vi "DefenderPenalty.vi"(6 "N atacantes":u32[](array[numeric]), 10 "Total de n \natacantes":i32, 11 "Robot in":T1={"id"=0, "function"=enum."Attacker", "x"=0.0, "y"=0.0, "orientation"=0.0, "v_tangent"=0.0, "v_normal"=0.0, "v_ang"=0.0, "kick_x"=0.0, "kick_z"=0.0, "dribble"=FALSE, "Timestamp"=timestamp(0 s since 1904-01-01), "estimatives"={"est_v_tangent"=0.0, "est_v_normal"=0.0, "est_vx"=0.0, "est_vy"=0.0, "Pos Robot Est"=[]}, "dest_x_kick"=0.0, "dest_y_kick"=0.0, "Gap Coord"=[], "States"=enum."GoToTangent", "Path "=[], "Path  Smooth"=[], "Dest"=[]}) -> (3 "Robot out":T1={"id"=0, "function"=enum."Attacker", "x"=0.0, "y"=0.0, "orientation"=0.0, "v_tangent"=0.0, "v_normal"=0.0, "v_ang"=0.0, "kick_x"=0.0, "kick_z"=0.0, "dribble"=FALSE, "Timestamp"=timestamp(0 s since 1904-01-01), "estimatives"={"est_v_tangent"=0.0, "est_v_normal"=0.0, "est_vx"=0.0, "est_vy"=0.0, "Pos Robot Est"=[]}, "dest_x_kick"=0.0, "dest_y_kick"=0.0, "Gap Coord"=[], "States"=enum."GoToTangent", "Path "=[], "Path  Smooth"=[], "Dest"=[]})   [LabVIEW 2017]
uses:
  Core/AI Robot.ctl
  Functions Enum.ctl
  AttackerStates.ctl
  Path Planning/RRT/PathDests.ctl
  Path Planning/RRT/PathDest.ctl
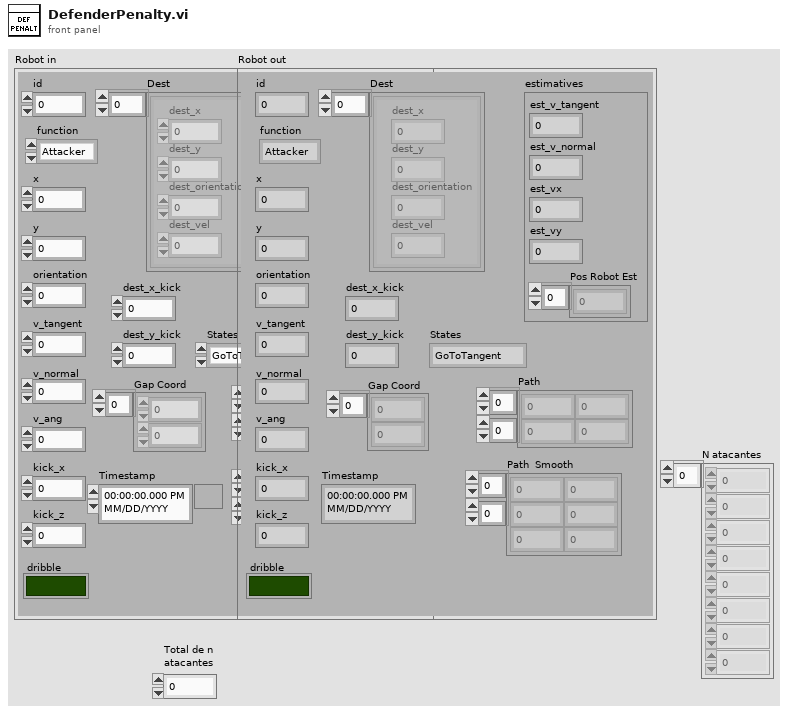
[diagram p1: front panel]
types:
  T1 = typedef "AI Robot.ctl" = cluster{"id":u32, "function":T2, "x":dbl, "y":dbl, "orientation":dbl, "v_tangent":dbl, "v_normal":dbl, "v_ang":dbl, "kick_x":dbl, "kick_z":dbl, "dribble":bool, "Timestamp":timestamp, "estimatives":cluster{"est_v_tangent":dbl, "est_v_normal":dbl, "est_vx":dbl, "est_vy":dbl, "Pos Robot Est":dbl[]}, "dest_x_kick":dbl, "dest_y_kick":dbl, "Gap Coord":dbl[], "States":T3, "Path ":dbl[][], "Path  Smooth":dbl[][], "Dest":T4}
  T2 = typedef "Functions Enum.ctl" = enum16{"Attacker", "Goalie", "Defender", "Striker", "Goto 0", "Dummy", "Kicker", "ZigZag"}
  T3 = typedef "AttackerStates.ctl" = enum16{"Pass", "GoToTangent", "BallGetting", "GoToKick", ""}
  T4 = typedef "PathDests.ctl" = T5[]
  T5 = typedef "PathDest.ctl" = cluster{"dest_x":dbl, "dest_y":dbl, "dest_orientation":dbl, "dest_vel":dbl}
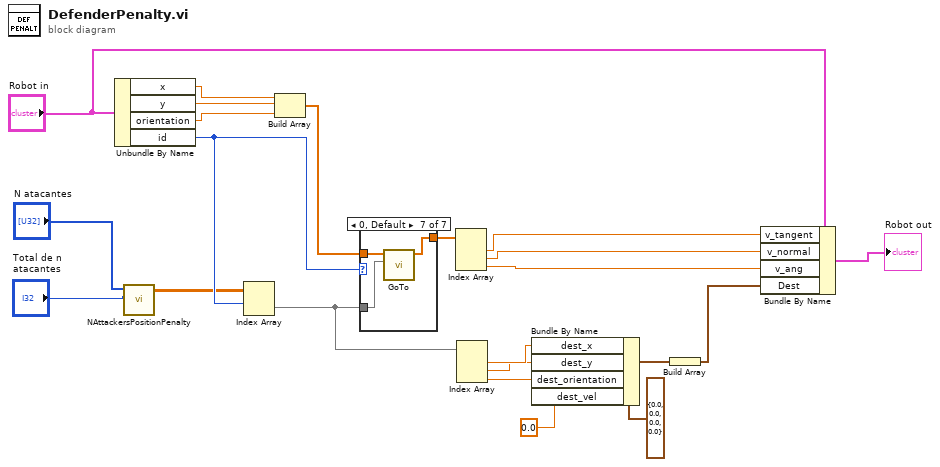
[diagram p0: block diagram]
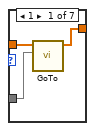
[diagram p2: hidden frame]
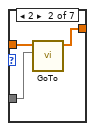
[diagram p3: hidden frame]
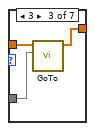
[diagram p4: hidden frame]
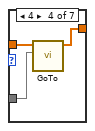
[diagram p5: hidden frame]
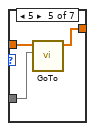
[diagram p6: hidden frame]
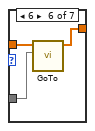
[diagram p7: hidden frame]
diagram:
  n1 = Unbundle By Name("Robot in") -> ("x"=w22:dbl, "y"=w21:dbl, "orientation"=w20:dbl, "id"=w12:u32)
  n2 = call "NAttackersPositionPenalty.vi"("N atacantes"="N atacantes", "Total de n \natacantes"="Total de n \natacantes") -> ("Posição dos não atacantes\ndurante o penalte"=w11:dbl[][])  [unwired: 8 in]
  n3 = Index Array(array=w11, index (row)=w12) -> (element=w8:dbl[])  [unwired: 1 in]
  n4 = Build Array(w22, w21, w20) -> (w19:dbl[])
  n5 = case shown="0, Default" w12 {
    tunnel: w19 -> [w25 w28 w31 w34 w37 w40 w43]
    tunnel: [w24 w27 w30 w33 w36 w39 w42] -> w18
    tunnel: w8 -> [w23 w26 w29 w32 w35 w38 w41]
    frame 1 {
      n6 = call "GoTo.vi"("Target"=w23, "Position"=w25) -> ("Output\nVelocity"=w24:dbl[])  [unwired: 8 in, 1 out]
    }
    frame 2 {
      n7 = call "GoTo.vi"("Target"=w26, "Position"=w28) -> ("Output\nVelocity"=w27:dbl[])  [unwired: 8 in, 1 out]
    }
    frame 3 {
      n8 = call "GoTo.vi"("Target"=w29, "Position"=w31) -> ("Output\nVelocity"=w30:dbl[])  [unwired: 8 in, 1 out]
    }
    frame 4 {
      n9 = call "GoTo.vi"("Target"=w32, "Position"=w34) -> ("Output\nVelocity"=w33:dbl[])  [unwired: 8 in, 1 out]
    }
    frame 5 {
      n10 = call "GoTo.vi"("Target"=w35, "Position"=w37) -> ("Output\nVelocity"=w36:dbl[])  [unwired: 8 in, 1 out]
    }
    frame 6 {
      n11 = call "GoTo.vi"("Target"=w38, "Position"=w40) -> ("Output\nVelocity"=w39:dbl[])  [unwired: 8 in, 1 out]
    }
    frame 0, Default {
      n12 = call "GoTo.vi"("Target"=w41, "Position"=w43) -> ("Output\nVelocity"=w42:dbl[])  [unwired: 8 in, 1 out]
    }
  }
  n13 = Index Array(array=w18) -> (element #1=w16:dbl, element #2=w15:dbl, element #3=w14:dbl)  [unwired: 3 in]
  n14 = Index Array(array=w8) -> (element #1=w3:dbl, element #2=w2:dbl, element #3=w1:dbl)  [unwired: 3 in]
  n15 = Bundle By Name(cluster=T5 {"dest_x"=0.0, "dest_y"=0.0, "dest_orientation"=0.0, "dest_vel"=0.0} ("Dest"), "dest_x"=w3, "dest_y"=w2, "dest_orientation"=w1, "dest_vel"=0.0) -> (w6:T5)
  n16 = Build Array(w6) -> (w4:T5[])
  n17 = Bundle By Name(cluster="Robot in", "v_tangent"=w16, "v_normal"=w15, "v_ang"=w14, "Dest"=w4) -> (→"Robot out":T1)
